vi "Open Account.vi"() -> (0 "错误输出":errorcluster, 3 "帐户信息":T1)   [LabVIEW 2012]
uses:
  Account Info.ctl
  Stop.vi
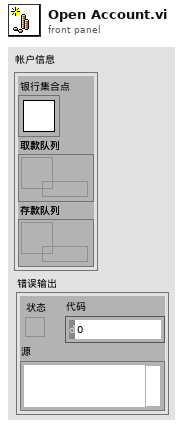
[diagram p1: front panel]
types:
  T1 = typedef "Account Info.ctl" = cluster{"银行集合点":T2, "取款队列":refnum<queue>, "存款队列":refnum<queue>}
  T2 = typedef "Rendezvous RefNum" = refnum<k1>
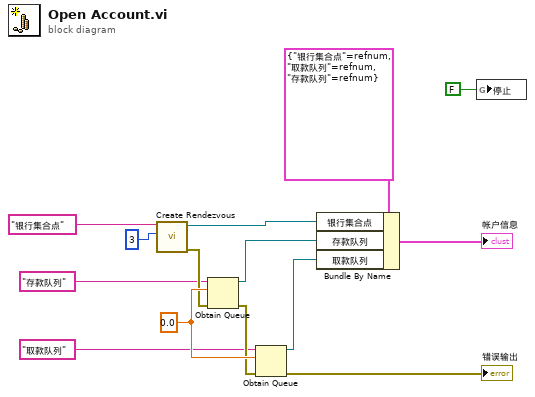
[diagram p0: block diagram]
diagram:
  w13 = 0.0
  n1 = call <vilib>:"Create Rendezvous.vi"("size (2)"=3 ("大小(2)"), "name (unnamed)"="银行集合点" ("名称（未命名）")) -> ("error out"=w12:errorcluster, "rendezvous"=w14:T2)  [unwired: 3 in, 1 out]
  n2 = Obtain Queue ("获取队列引用")(name (unnamed)="存款队列" ("名称（未命名）"), element data type=w13, error in (no error)=w12) -> (queue out=w10:refnum<queue>, error out=w11:errorcluster)  [unwired: 2 in, 1 out]
  n3 = Obtain Queue ("获取队列引用")(name (unnamed)="取款队列" ("名称（未命名）"), element data type=w13, error in (no error)=w11) -> (queue out=w9:refnum<queue>, error out=→"错误输出":errorcluster)  [unwired: 2 in, 1 out]
  n4 = Bundle By Name ("按名称捆绑")(cluster=T1 {"银行集合点"=refnum, "取款队列"=refnum, "存款队列"=refnum} ("簇"), "银行集合点"=w14, "存款队列"=w10, "取款队列"=w9) -> (→"帐户信息":T1)
  n5 = global write "Stop.vi" "停止"(FALSE ("停止")) -> ()
